vi "Settings_Config.vi"(11 "DataCluster in":T1={"Core"={"Current VI Reference"=refnum, "Close Panel on Exit?"=FALSE, "Exit"=FALSE}, "Connections"={"cDAQ"={"Task"="", "Connected"=FALSE, "Active"=FALSE}, "Camera"={"Session"="", "Connected"=FALSE, "Active"=FALSE}}, "Data Acquisition"={"Setup"={"Label"="", "Operator"="", "Notes"="", "TempGrad"=1.0, "TargetTemp"=1.0}, "Camera"={"Image"=refnum, "Save Image"=refnum}, "Thermistor"={"Sample Size"=0, "Calibration"={"B0.100"=[], "R25"=[], "V_S"=5.0, "R_S"=100.0}}, "Queue"={"Size"=1, "Queue"=refnum}, "Sample Rate"=1, "Active"=FALSE, "Ready"=FALSE}} {"Data Acquisition"."Thermistor"."Calibration"."R_S" min=0.1 max=1000.0 format="%#_g kOhm"; "Data Acquisition"."Thermistor"."Calibration"."V_S" min=5.0 max=48.0 format="%#_g V"; "Data Acquisition"."Thermistor"."Calibration"."R25" min=0.1 max=1000.0 format="%#_g kOhm"; "Data Acquisition"."Thermistor"."Calibration"."B0.100" min=100.0 max=10000.0 format="%#_g K"; "Data Acquisition"."Thermistor"."Sample Size" min=1 max=200; "Data Acquisition"."Sample Rate" min=1 max=240; "Data Acquisition"."Queue"."Size" min=1 max=200; "Data Acquisition"."Setup"."TargetTemp" min=-30.0 max=30.0 step=0.5 format="%#_g °C"; "Data Acquisition"."Setup"."TempGrad" min=-100.0 max=100.0 step=0.1 format="%#_g °C/min"}) -> (3 "DataCluster out":T1={"Core"={"Current VI Reference"=refnum, "Close Panel on Exit?"=FALSE, "Exit"=FALSE}, "Connections"={"cDAQ"={"Task"="", "Connected"=FALSE, "Active"=FALSE}, "Camera"={"Session"="", "Connected"=FALSE, "Active"=FALSE}}, "Data Acquisition"={"Setup"={"Label"="", "Operator"="", "Notes"="", "TempGrad"=1.0, "TargetTemp"=1.0}, "Camera"={"Image"=refnum, "Save Image"=refnum}, "Thermistor"={"Sample Size"=0, "Calibration"={"B0.100"=[], "R25"=[], "V_S"=5.0, "R_S"=100.0}}, "Queue"={"Size"=1, "Queue"=refnum}, "Sample Rate"=1, "Active"=FALSE, "Ready"=FALSE}} {"Data Acquisition"."Thermistor"."Calibration"."R_S" min=0.1 max=1000.0 format="%#_g kOhm"; "Data Acquisition"."Thermistor"."Calibration"."V_S" min=5.0 max=48.0 format="%#_g V"; "Data Acquisition"."Thermistor"."Calibration"."R25" min=0.1 max=1000.0 format="%#_g kOhm"; "Data Acquisition"."Thermistor"."Calibration"."B0.100" min=100.0 max=10000.0 format="%#_g K"; "Data Acquisition"."Thermistor"."Sample Size" min=1 max=200; "Data Acquisition"."Sample Rate" min=1 max=240; "Data Acquisition"."Queue"."Size" min=1 max=200; "Data Acquisition"."Setup"."TargetTemp" min=-30.0 max=30.0 step=0.5 format="%#_g °C"; "Data Acquisition"."Setup"."TempGrad" min=-100.0 max=100.0 step=0.1 format="%#_g °C/min"})   [LabVIEW 2020]
uses:
  DataCluster.ctl
  <vilib>/userDefined/High Color/IMAQdx.ctl
  <vilib>/vision/Image Controls.llb/IMAQ Image.ctl
panel:
  in  "Sample Rate":i32=1 min=1 max=240 step=1 format="%.0f Samples/min"
  in  "Sample Size":i32=1 min=1 max=200 step=1
  in  "Buffer Size":i32=1 min=1 max=300 step=1
  in  "Target Temperature":dbl=1.0 min=-30.0 max=30.0 step=0.5 format="%#_g °C"
  in  "OK":bool
  in  "Cancel":bool
  in  "Temperature Gradient":dbl=1.0 min=-100.0 max=100.0 step=0.1 format="%#_g °C/min"
  in  "Notes":string
  in  "Operator":string
  in  "Label":string
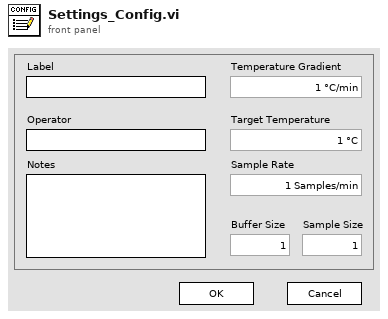
[diagram p1: front panel]
types:
  T1 = typedef "DataCluster.ctl" = cluster{"Core":cluster{"Current VI Reference":refnum<vi>, "Close Panel on Exit?":bool, "Exit":bool}, "Connections":cluster{"cDAQ":cluster{"Task":refnum<k21>, "Connected":bool, "Active":bool}, "Camera":cluster{"Session":T2, "Connected":bool, "Active":bool}}, "Data Acquisition":cluster{"Setup":cluster{"Label":string, "Operator":string, "Notes":string, "TempGrad":dbl, "TargetTemp":dbl}, "Camera":cluster{"Image":T3, "Save Image":T3}, "Thermistor":cluster{"Sample Size":i32, "Calibration":cluster{"B0.100":dbl[], "R25":dbl[], "V_S":dbl, "R_S":dbl}}, "Queue":cluster{"Size":i32, "Queue":refnum<queue>}, "Sample Rate":i32, "Active":bool, "Ready":bool}}
  T2 = typedef "IMAQdx.ctl" = refnum<k21>
  T3 = typedef "IMAQ Image.ctl" = refnum<image>
  T4 = cluster{"Label":string, "Operator":string, "Notes":string, "TempGrad":dbl, "TargetTemp":dbl}
  T5 = enum8{"Enabled", "Disabled", "Disabled and Grayed Out"}
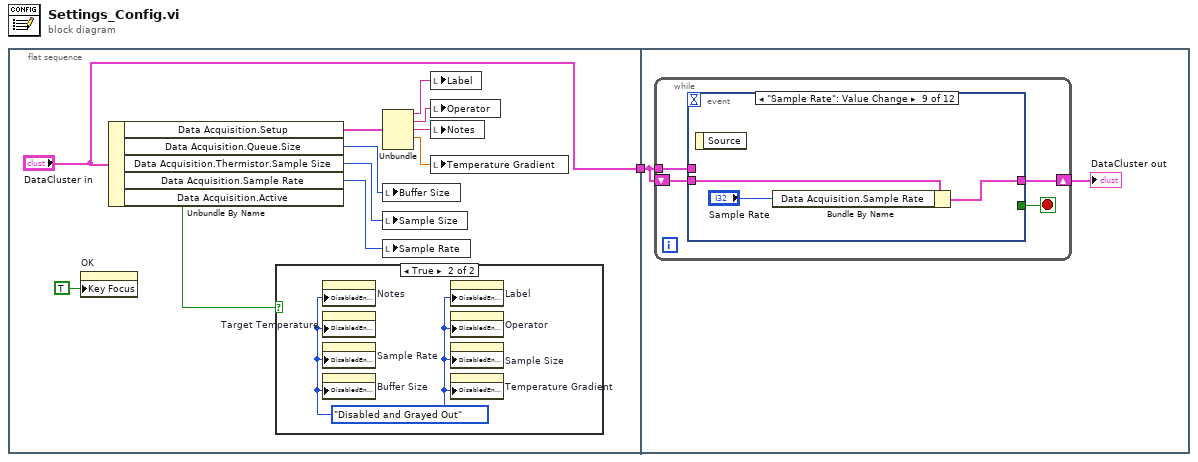
[diagram p0: block diagram]
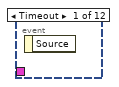
[diagram p3: hidden frame]
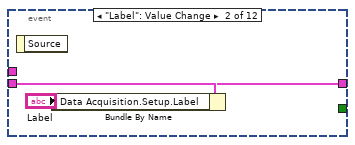
[diagram p4: hidden frame]
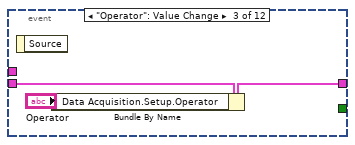
[diagram p5: hidden frame]
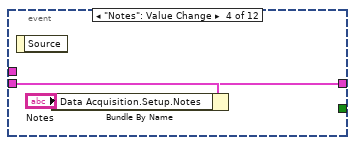
[diagram p6: hidden frame]
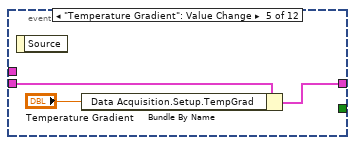
[diagram p7: hidden frame]
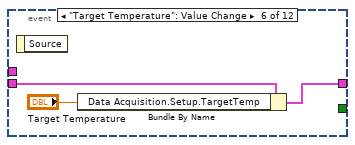
[diagram p8: hidden frame]
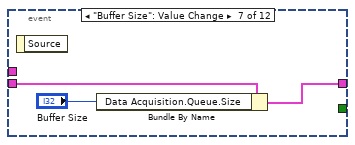
[diagram p9: hidden frame]
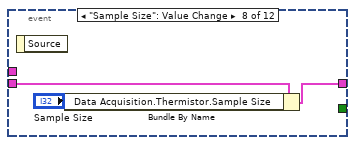
[diagram p10: hidden frame]
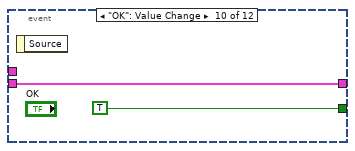
[diagram p11: hidden frame]
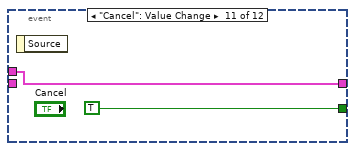
[diagram p12: hidden frame]
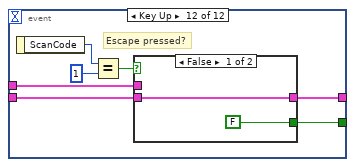
[diagram p13: hidden frame]
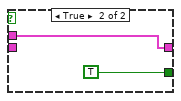
[diagram p14: hidden frame]
diagram:
  n1 = flat-sequence {
    tunnel: ["DataCluster in"] -> w1
    tunnel: w1 -> [w15]
    frame #0 {
      n2 = property on="OK" class="Bool"("Key Focus"=TRUE) -> ()  [unwired: 2 in, 2 out]
      n3 = Unbundle By Name("DataCluster in") -> ("Data Acquisition.Setup"=w12:T4, "Data Acquisition.Queue.Size"=w7:i32, "Data Acquisition.Thermistor.Sample Size"=w4:i32, "Data Acquisition.Sample Rate"=w3:i32, "Data Acquisition.Active"=w2:bool)
      n4 = case shown="True" w2 {
        frame False {
        }
        frame True {
          w13 = T5."Disabled and Grayed Out" ("Disabled")
          n5 = property on="Notes" class="Str"("DisabledEnum"=w13) -> ()  [unwired: 2 in, 2 out]
          n6 = property on="Target Temperature" class="DigNum (strict)"("DisabledEnum"=w13) -> ()  [unwired: 2 in, 2 out]
          n7 = property on="Sample Rate" class="DigNum (strict)"("DisabledEnum"=w13) -> ()  [unwired: 2 in, 2 out]
          n8 = property on="Buffer Size" class="DigNum (strict)"("DisabledEnum"=w13) -> ()  [unwired: 2 in, 2 out]
          n9 = property on="Label" class="Str"("DisabledEnum"=w13) -> ()  [unwired: 2 in, 2 out]
          n10 = property on="Operator" class="Str"("DisabledEnum"=w13) -> ()  [unwired: 2 in, 2 out]
          n11 = property on="Sample Size" class="DigNum (strict)"("DisabledEnum"=w13) -> ()  [unwired: 2 in, 2 out]
          n12 = property on="Temperature Gradient" class="DigNum (strict)"("DisabledEnum"=w13) -> ()  [unwired: 2 in, 2 out]
        }
      }
      n13 = Unbundle(w12) -> ("Label"=w11:string, "Operator"=w6:string, "Notes"=w5:string, "TempGrad"=w10:dbl)  [unwired: 1 out]
      n14 = local write "Buffer Size"(w7) -> ()
      n15 = local write "Sample Size"(w4) -> ()
      n16 = local write "Sample Rate"(w3) -> ()
      n17 = local write "Label"(w11) -> ()
      n18 = local write "Operator"(w6) -> ()
      n19 = local write "Notes"(w5) -> ()
      n20 = local write "Temperature Gradient"(w10) -> ()
    }
    frame #1 {
      n21 = while {
        shift-right: [w19] -> w14
        shift-left: w15 -> [w18]
        tunnel: w15 -> [w17]
        stop <- w16 stop-if-true
        n22 = event shown="[8] \"Sample Rate\": Value Change" {
          selector: _ -> [_ _ _ _ _ _ _ _ _ _ _ _]
          dyn-events: _ -> [_ _ _ _ _ _ _ _ _ _ _ _]
          timeout: _ -> [_ _ _ _ _ _ _ _ _ _ _ _]
          tunnel: w18 -> [_ w22 w25 w28 w31 w34 w37 w40 w43 w45 _ w48]
          tunnel: [_ w21 w24 w27 w30 w33 w36 w39 w42 w45 w47 w50] -> w19
          tunnel: w17 -> [_ _ _ _ _ _ _ _ _ _ w47 w49]
          tunnel: [_ _ _ _ _ _ _ _ _ TRUE TRUE w54] -> w16
          event Timeout {
            n23 = event-data() -> ()  [unwired: 1 in, 1 out]
          }
          event "Label": Value Change {
            n24 = event-data() -> ()  [unwired: 1 in, 1 out]
            n25 = Bundle By Name(cluster=w22, "Data Acquisition.Setup.Label"="Label") -> (w21:T1)
          }
          event "Operator": Value Change {
            n26 = event-data() -> ()  [unwired: 1 in, 1 out]
            n27 = Bundle By Name(cluster=w25, "Data Acquisition.Setup.Operator"="Operator") -> (w24:T1)
          }
          event "Notes": Value Change {
            n28 = event-data() -> ()  [unwired: 1 in, 1 out]
            n29 = Bundle By Name(cluster=w28, "Data Acquisition.Setup.Notes"="Notes") -> (w27:T1)
          }
          event "Temperature Gradient": Value Change {
            n30 = event-data() -> ()  [unwired: 1 in, 1 out]
            n31 = Bundle By Name(cluster=w31, "Data Acquisition.Setup.TempGrad"="Temperature Gradient") -> (w30:T1)
          }
          event "Target Temperature": Value Change {
            n32 = event-data() -> ()  [unwired: 1 in, 1 out]
            n33 = Bundle By Name(cluster=w34, "Data Acquisition.Setup.TargetTemp"="Target Temperature") -> (w33:T1)
          }
          event "Buffer Size": Value Change {
            n34 = event-data() -> ()  [unwired: 1 in, 1 out]
            n35 = Bundle By Name(cluster=w37, "Data Acquisition.Queue.Size"="Buffer Size") -> (w36:T1)
          }
          event "Sample Size": Value Change {
            n36 = event-data() -> ()  [unwired: 1 in, 1 out]
            n37 = Bundle By Name(cluster=w40, "Data Acquisition.Thermistor.Sample Size"="Sample Size") -> (w39:T1)
          }
          event "Sample Rate": Value Change {
            n38 = event-data() -> ()  [unwired: 1 in, 1 out]
            n39 = Bundle By Name(cluster=w43, "Data Acquisition.Sample Rate"="Sample Rate") -> (w42:T1)
          }
          event "OK": Value Change {
            n40 = event-data() -> ()  [unwired: 1 in, 1 out]
          }
          event "Cancel": Value Change {
            n41 = event-data() -> ()  [unwired: 1 in, 1 out]
          }
          event Key Up {
            # "Escape pressed?"
            n42 = event-data() -> ("ScanCode"=w53:i16)  [unwired: 1 in]
            n43 = Equal?(x=w53, y=i16 1) -> (x = y?=w51:bool)
            n44 = case shown="False" w51 {
              tunnel: [FALSE TRUE] -> w54
              tunnel: [w56 w57] -> w50
              tunnel: w49 -> [_ w57]
              tunnel: w48 -> [w56 _]
              frame False {
              }
              frame True {
              }
            }
          }
        }
      }
      "DataCluster out" <- w14
    }
  }
